vi "matlab_for_edges.vi"(8 "dmd pattern num":dbl, 11 "exposure_time(ms)":dbl) -> (0 "exposure time":dbl, 1 "sample num":dbl, 2 "DO signal":dbl[][](array[numeric]), 3 "sample rate":dbl, 5 "dmd_picture_time":dbl)   [LabVIEW 2019]
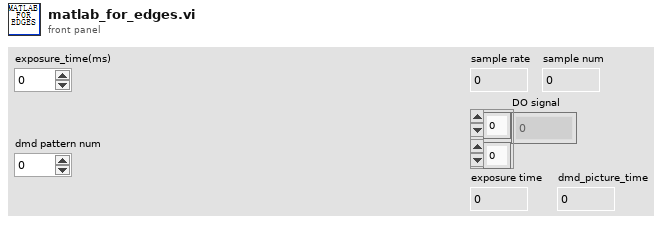
[diagram p1: front panel]
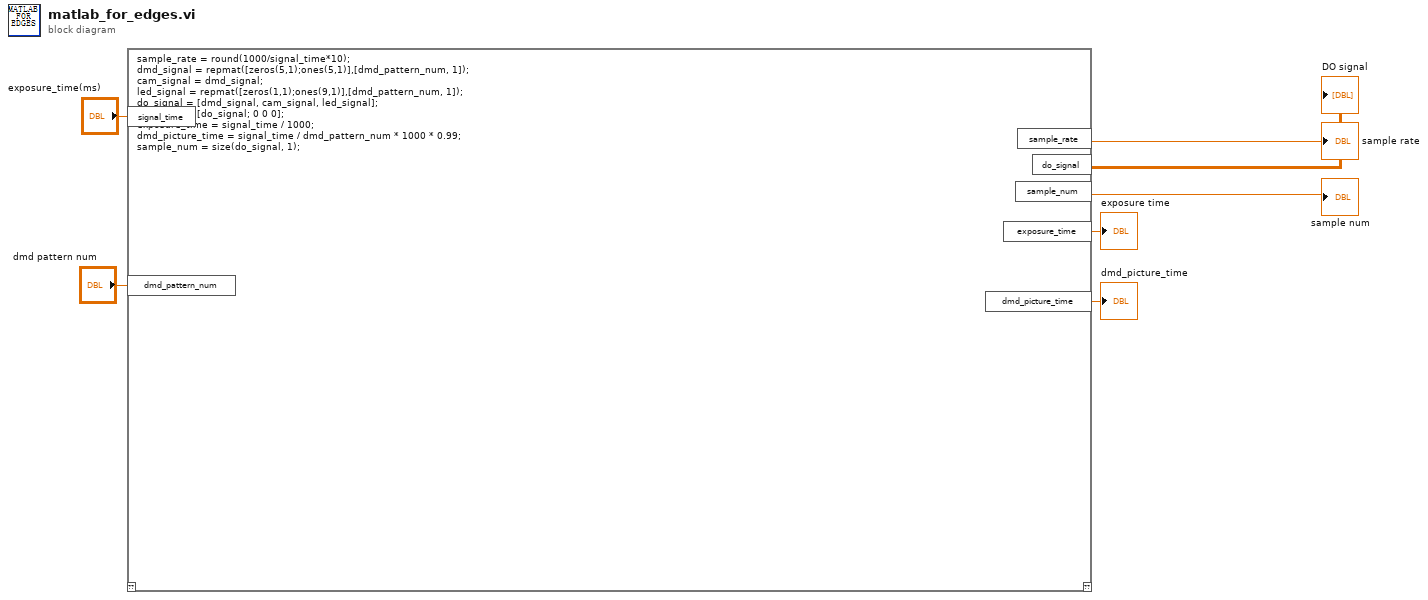
[diagram p0: block diagram]
diagram:
  n1 = script code="sample_rate = round(1000/signal_time*10);\ndmd_signal = repmat([zeros(5,1);ones(5,1)],[dmd_pattern_num, 1]);\ncam_signal = dmd_signal;\nled_signal = repmat([zeros(1,1);ones(9,1)],[dmd_pattern_num, 1]);\ndo_signal = [dmd_signal, cam_signal, led_signal];\ndo_signal = [do_signal; 0 0 0];\nexposure_time = signal_time / 1000;\ndmd_picture_time = signal_time / dmd_pattern_num * 1000 * 0.99;\nsample_num = size(do_signal, 1);"("signal_time"="exposure_time(ms)", "dmd_pattern_num"="dmd pattern num") -> ("do_signal"=→"DO signal":dbl[][], "sample_rate"=→"sample rate":dbl, "sample_num"=→"sample num":dbl, "exposure_time"=→"exposure time":dbl, "dmd_picture_time"=→"dmd_picture_time":dbl)  [unwired: 1 in, 1 out]
